vi "main.vi"() -> ()   [LabVIEW 2017]
uses:
  <vilib>/Instr/_visa.llb/VISA Set IO Buffer Mask.ctl
  <vilib>/Instr/_visa.llb/VISA Configure Serial Port (Instr).vi
  <vilib>/Analysis/NI_AALBase.lvlib
panel:
  in  "保存按钮":bool
  out "standard deviation":dbl caption="标准差" format="%#_2f"
  out "mean":dbl caption="均值" format="%#_7f"
  out "波形图表":dbl(graph)
  in  "配置Pcap":bool
  out "发送字符数":dbl
  in  "清空按钮":bool
  in  "timeout (10sec)":u32=100 caption="读取超时"
  in  "baud rate (9600)":u32=115200 caption="波特率"
  in  "VISA resource name":refnum<visa-resource-name> caption="串口号"
  in  "读取字节数":u32=1000
  out "未知的参数":string
  in  "参数数组":string[][](array[string])=[[""]]
  in  "发送自定义参数按钮":bool
  in  "自定义参数":string
  out "远程消息":string
  out "长度":i32=440
  out "连接状态":bool
  in  "查询次数":dbl
  in  "采集开关":bool
  in  "待处理数据":string
  # "最近10个数据统计值"
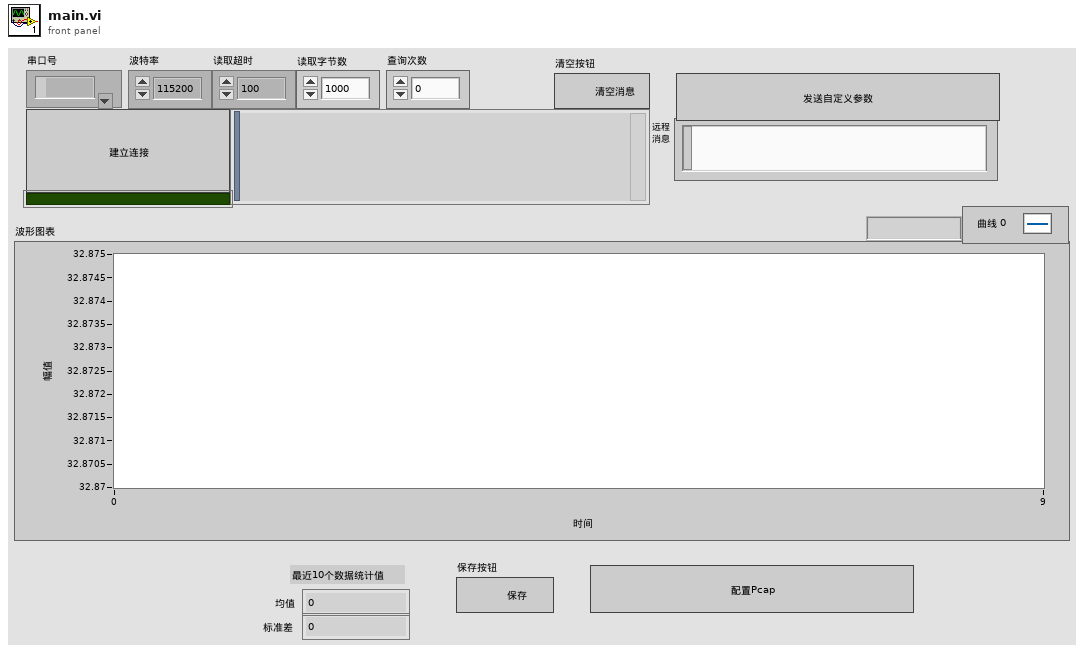
[diagram p1: front panel]
types:
  T1 = typedef "VISA Set IO Buffer Mask.ctl" = u16
  T2 = enum16{"big-endian, network order", "native, host order", "little-endian"}
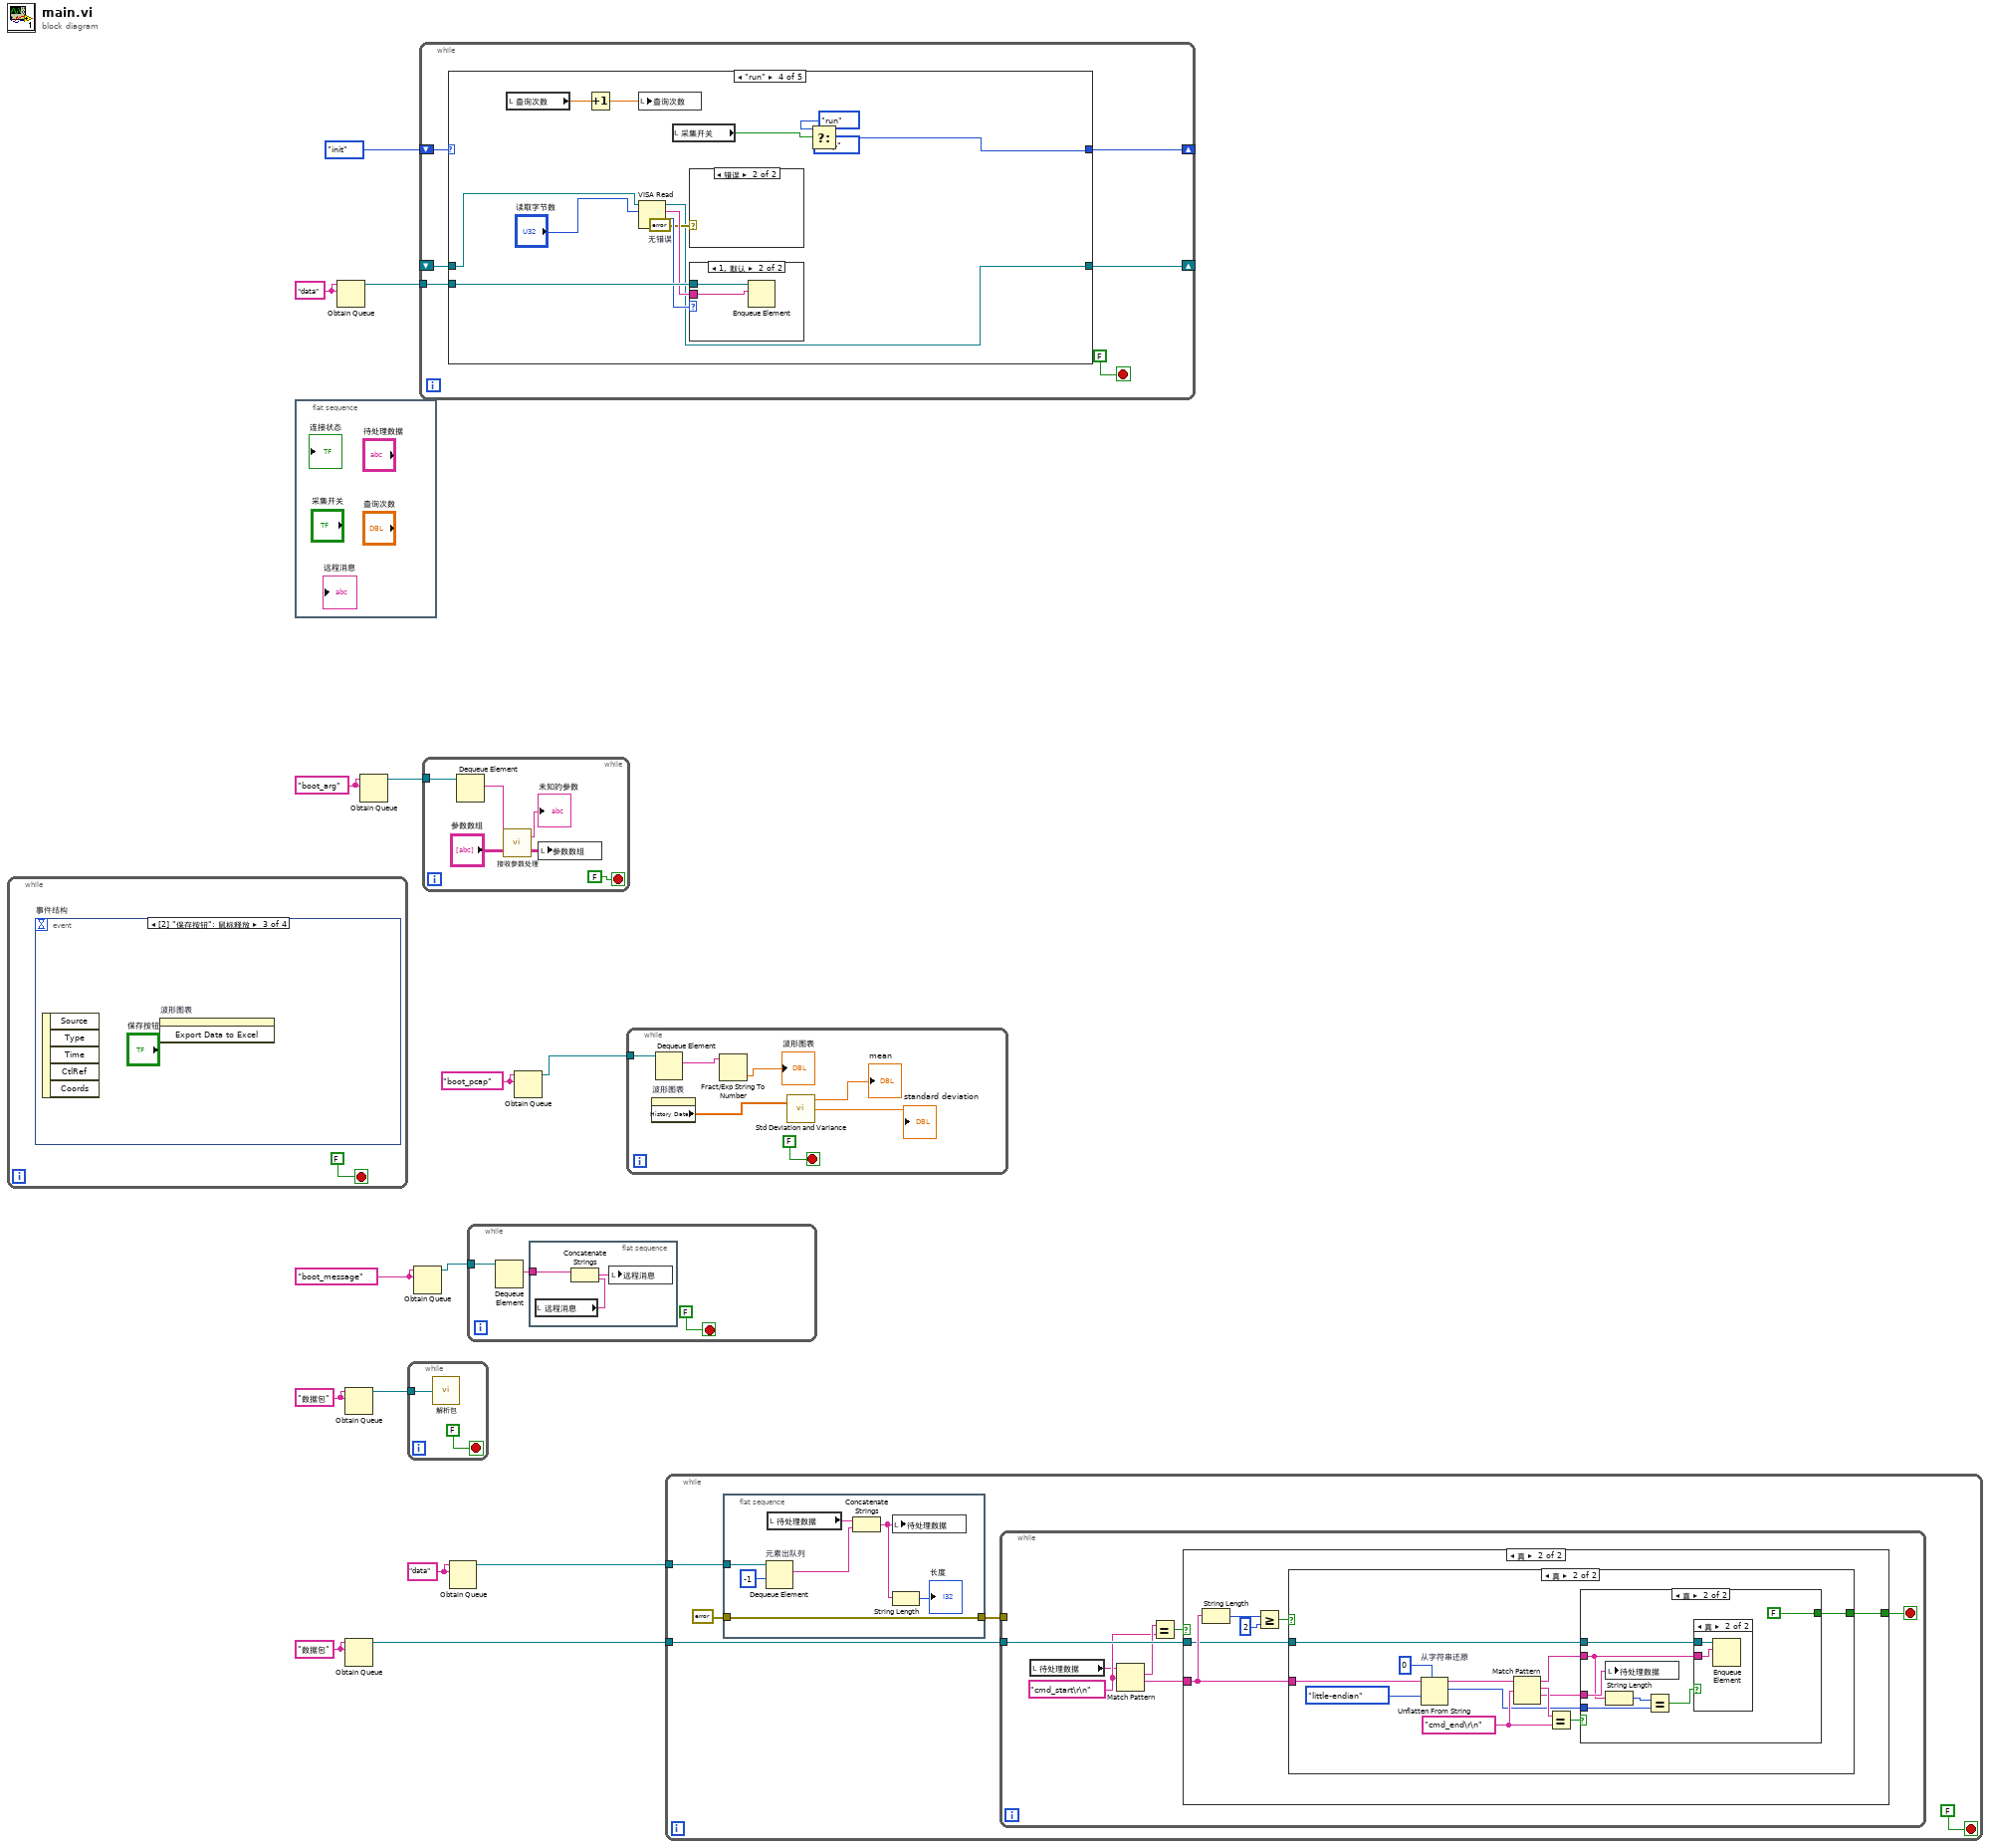
[diagram p0: block diagram]
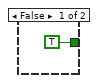
[diagram p2: hidden frame]
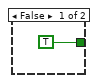
[diagram p3: hidden frame]
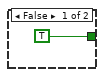
[diagram p4: hidden frame]
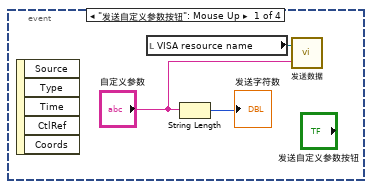
[diagram p6: hidden frame]
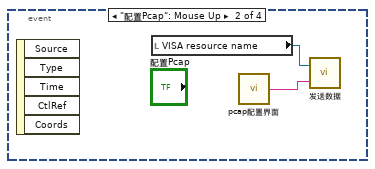
[diagram p7: hidden frame]
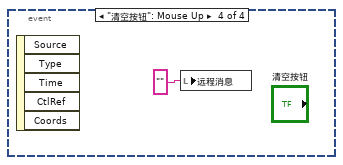
[diagram p8: hidden frame]
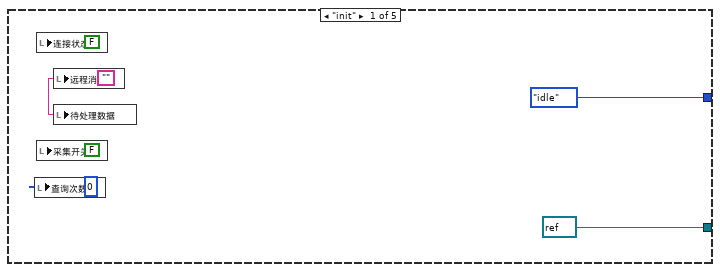
[diagram p9: hidden frame]
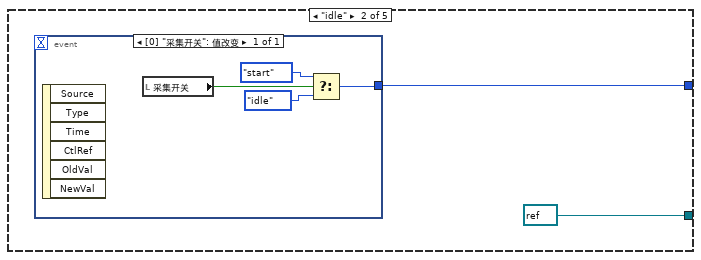
[diagram p10: hidden frame]
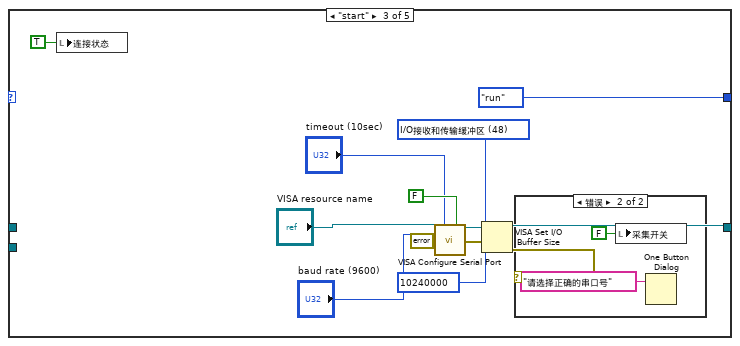
[diagram p11: hidden frame]
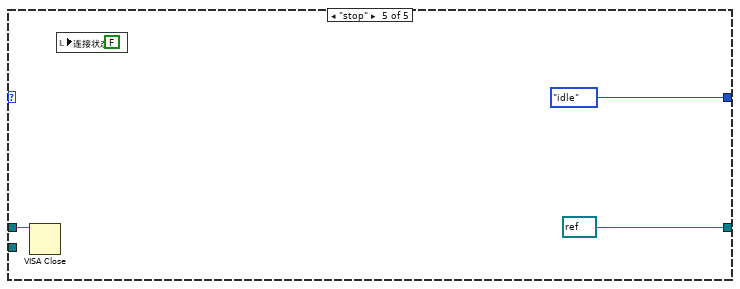
[diagram p15: hidden frame]
diagram:
  w2 = "boot_pcap" ("名称（未命名）")
  w4 = "boot_arg" ("名称（未命名）")
  w5 = "数据包" ("名称（未命名）")
  w8 = "boot_message" ("名称（未命名）")
  w11 = "数据包" ("名称（未命名）")
  w13 = "data" ("名称（未命名）")
  w15 = "data" ("名称（未命名）")
  n1 = while {
    stop <- FALSE stop-if-true
    n2 = event "事件结构" shown="[2] \"保存按钮\": 鼠标释放" {
      selector: _ -> [_ _ _ _]
      dyn-events: _ -> [_ _ _ _]
      timeout: _ -> [_ _ _ _]
      event "发送自定义参数按钮": Mouse Up {
        n3 = event-data() -> ()  [unwired: 1 in, 5 out]
        n4 = local read "VISA resource name"() -> (w19:refnum<visa-resource-name>)
        n5 = String Length(string="自定义参数") -> (length=→"发送字符数":i32)
        n6 = call "发送数据.vi"("发送数据"="自定义参数", "VISA资源名称"=w19) -> ()  [unwired: 1 in]
      }
      event "配置Pcap": Mouse Up {
        n7 = event-data() -> ()  [unwired: 1 in, 5 out]
        n8 = local read "VISA resource name"() -> (w20:refnum<visa-resource-name>)
        n9 = call "pcap配置界面.vi"() -> ("电子表格字符串"=w21:string)
        n10 = call "发送数据.vi"("发送数据"=w21, "VISA资源名称"=w20) -> ()  [unwired: 1 in]
      }
      event "保存按钮": Mouse Up {
        n11 = event-data() -> ()  [unwired: 1 in, 5 out]
        n12 = invoke on="波形图表" class="WFChart (严格)" method="Export Data to Excel"() -> ()  [unwired: 3 in, 3 out]
      }
      event "清空按钮": Mouse Up {
        n13 = event-data() -> ()  [unwired: 1 in, 5 out]
        n14 = local write "远程消息"("" ("远程消息")) -> ()
      }
    }
  }
  n15 = flat-sequence {
    frame #0 {
    }
  }
  n16 = Obtain Queue(name (unnamed)=w13, element data type=w13) -> (queue out=w12:refnum<queue>)  [unwired: 3 in, 2 out]
  n17 = Obtain Queue(name (unnamed)=w5, element data type=w5) -> (queue out=w6:refnum<queue>)  [unwired: 3 in, 2 out]
  n18 = Obtain Queue(name (unnamed)=w11, element data type=w11) -> (queue out=w10:refnum<queue>)  [unwired: 3 in, 2 out]
  n19 = Obtain Queue(name (unnamed)=w4, element data type=w4) -> (queue out=w3:refnum<queue>)  [unwired: 3 in, 2 out]
  n20 = while {
    tunnel: w6 -> [w23]
    stop <- FALSE stop-if-true
    n21 = call "解析包.vi"("数据包队列名称"=w23) -> ()  [unwired: 1 out]
  }
  n22 = Obtain Queue(name (unnamed)=w8, element data type=w8) -> (queue out=w7:refnum<queue>)  [unwired: 3 in, 2 out]
  n23 = while {
    shift-right: [w29] -> _
    shift-left: enum16{"start", "run", "stop", "idle", "init"}."init" -> [w30]
    tunnel: w12 -> [w27]
    shift-right: [w25] -> _
    shift-left: _ -> [w26]
    stop <- FALSE stop-if-true
    n24 = case shown="\"run\"" w30 {
      tunnel: [enum16{"start", "run", "stop", "idle", "init"}."idle" w38 enum16{"start", "run", "stop", "idle"}."run" w68 enum16{"start", "run", "stop", "idle"}."idle"] -> w29
      tunnel: w27 -> [_ _ _ w62 _]
      tunnel: [refnum<visa-resource-name> refnum ("VISA resource name out") refnum<visa-resource-name> refnum ("VISA resource name out") w47 w57 refnum<visa-resource-name> refnum ("VISA resource name out")] -> w25
      tunnel: w26 -> [_ _ _ w58 w74]
      frame "init" {
        w34 = ""
        n25 = local write "查询次数"(u16 0 ("宽")) -> ()
        n26 = local write "连接状态"(FALSE) -> ()
        n27 = local write "采集开关"(FALSE ("采样开关")) -> ()
        n28 = local write "远程消息"(w34) -> ()
        n29 = local write "待处理数据"(w34) -> ()
      }
      frame "idle" {
        n30 = event shown="[0] \"采集开关\": 值改变" {
          selector: _ -> [_]
          dyn-events: _ -> [_]
          timeout: _ -> [_]
          tunnel: [w39] -> w38
          event "采集开关": Value Change {
            n31 = event-data() -> ()  [unwired: 1 in, 6 out]
            n32 = local read "采集开关"() -> (w42:bool)
            n33 = Select(t=enum16{"start", "run", "stop", "idle"}."start", s=w42, f=enum16{"start", "run", "stop", "idle"}."idle") -> (s? t:f=w39:enum16{"start", "run", "stop", "idle"})
          }
        }
      }
      frame "start" {
        w46 = T1 48 items=["I/O接收缓冲区"=16, "I/O传输缓冲区"=32, "I/O接收和传输缓冲区"=48] ("Mask")
        n34 = local write "连接状态"(TRUE ("连接状态")) -> ()
        n35 = call-poly "VISA Configure Serial Port"("VISA resource name"="VISA resource name", "timeout (10sec)"="timeout (10sec)", "Enable Termination\nChar (T)"=FALSE ("Enable Termination\nChar (T)"), "baud rate (9600)"="baud rate (9600)") -> ("VISA resource name out"=w48:refnum<visa-resource-name>)  [unwired: 10 in, 1 out]
        n36 = VISA Set I/O Buffer Size(VISA resource name=w48, mask (16)=w46, size (4096)=u32 10240000 ("大小(4096)"), error in (no error)=errorcluster {"status"=FALSE, "code"=0, "source"=""} ("错误输入（无错误）")) -> (VISA resource name out=w47:refnum<visa-resource-name>, error out=w43:errorcluster)
        n37 = case shown="错误" w43 {
          frame No Error {
          }
          frame Error {
            n38 = local write "采集开关"(FALSE ("采集开关")) -> ()
            n39 = One Button Dialog(message="请选择正确的串口号" ("消息")) -> ()  [unwired: 1 in, 1 out]
          }
        }
      }
      frame "run" {
        w63 = errorcluster {"status"=FALSE, "code"=0, "source"=""}  # 无错误
        n40 = local read "查询次数"() -> (w66:dbl)
        n41 = Increment(x=w66) -> (x+1=w65:dbl)
        n42 = local write "查询次数"(w65) -> ()
        n43 = VISA Read(VISA resource name=w58, byte count="读取字节数", error in (no error)=w63) -> (VISA resource name out=w57:refnum<visa-resource-name>, read buffer=w61:string, return count=w60:u32, error out=w59:errorcluster)
        n44 = local read "采集开关"() -> (w70:bool)
        n45 = case shown="错误" w59 {
          frame No Error {
          }
          frame Error {
          }
        }
        n46 = case shown="1, 默认" w60 {
          tunnel: w62 -> [_ w71]
          tunnel: w61 -> [_ w72]
          frame 0 {
          }
          frame 1, Default {
            n47 = Enqueue Element(queue=w71, element=w72) -> ()  [unwired: 2 in, 3 out]
          }
        }
        n48 = Select(t=enum16{"start", "run", "stop", "idle"}."run", s=w70, f=enum16{"start", "run", "stop", "idle"}."stop") -> (s? t:f=w68:enum16{"start", "run", "stop", "idle"})
      }
      frame "stop" {
        n49 = VISA Close(VISA resource name=w74) -> ()  [unwired: 1 in, 1 out]
        n50 = local write "连接状态"(FALSE ("连接状态")) -> ()
      }
    }
  }
  n51 = while {
    tunnel: w3 -> [w82]
    stop <- FALSE stop-if-true
    n52 = Dequeue Element(queue=w82) -> (element=w77:string)  [unwired: 2 in, 3 out]
    n53 = call "接收参数处理.vi"("输入参数数组"="参数数组", "参数字符串"=w77) -> ("输出参数数组"=w80:string[][], "未知的参数"=→"未知的参数":string)
    n54 = local write "参数数组"(w80) -> ()
  }
  n55 = Obtain Queue(name (unnamed)=w15, element data type=w15) -> (queue out=w9:refnum<queue>)  [unwired: 3 in, 2 out]
  n56 = while {
    tunnel: w7 -> [w85]
    stop <- FALSE stop-if-true
    n57 = Dequeue Element(queue=w85) -> (element=w83:string)  [unwired: 2 in, 3 out]
    n58 = flat-sequence {
      tunnel: w83 -> [w86]
      frame #0 {
        n59 = local read "远程消息"() -> (w88:string)
        n60 = Concatenate Strings(w86, w88) -> (w87:string)
        n61 = local write "远程消息"(w87) -> ()
      }
    }
  }
  n62 = Obtain Queue(name (unnamed)=w2, element data type=w2) -> (queue out=w1:refnum<queue>)  [unwired: 3 in, 2 out]
  n63 = while {
    tunnel: w1 -> [w95]
    stop <- FALSE stop-if-true
    n64 = property on="波形图表" class="WFChart (严格)"() -> ("History Data"=w89:dbl[])  [unwired: 2 in, 2 out]
    n65 = Dequeue Element(queue=w95) -> (element=w93:string)  [unwired: 2 in, 3 out]
    n66 = Fract/Exp String To Number(string=w93) -> (number=→"波形图表":dbl)  [unwired: 3 in, 1 out]
    n67 = call <vilib>:"Std Deviation and Variance.vi"("X"=w89) -> ("mean"=→"mean":dbl, "standard deviation"=→"standard deviation":dbl)  [unwired: 1 in, 1 out]
  }
  n68 = while {
    tunnel: w10 -> [w99]
    tunnel: w9 -> [w98]
    stop <- FALSE stop-if-true
    n69 = flat-sequence {
      tunnel: w98 -> [w107]
      tunnel: errorcluster {"status"=FALSE, "code"=0, "source"=""} ("错误常量") -> [w101]
      tunnel: [w101] -> w96
      frame #0 {
        n70 = Dequeue Element "元素出队列"(queue=w107, timeout in ms (-1)=-1 ("超时毫秒(-1)")) -> (element=w105:string)  [unwired: 1 in, 3 out]
        n71 = local read "待处理数据"() -> (w104:string)
        n72 = Concatenate Strings(w104, w105) -> (w106:string)
        n73 = local write "待处理数据"(w106) -> ()
        n74 = String Length(string=w106) -> (length=→"长度":i32)
      }
    }
    n75 = while {
      tunnel: w99 -> [w112]
      tunnel: w96 -> [_]
      stop <- w108 stop-if-true
      w110 = "cmd_start\r\n" ("正则表达式")
      n76 = local read "待处理数据"() -> (w109:string)
      n77 = Match Pattern(string=w109, regular expression=w110) -> (match substring=w111:string, after substring=w113:string)  [unwired: 1 in, 2 out]
      n78 = Equal?(x=w111, y=w110) -> (x = y?=w114:bool)
      n79 = case shown="真" w114 {
        tunnel: w113 -> [_ w118]
        tunnel: w112 -> [_ w117]
        tunnel: [TRUE w116] -> w108
        frame False {
        }
        frame True {
          n80 = String Length(string=w118) -> (length=w121:i32)
          n81 = Greater Or Equal?(x=w121, y=2) -> (x >= y?=w119:bool)
          n82 = case shown="真" w119 {
            tunnel: w118 -> [_ w132]
            tunnel: w117 -> [_ w126]
            tunnel: [TRUE w124] -> w116
            frame False {
            }
            frame True {
              w129 = "cmd_end\r\n" ("结束码")
              n83 = Unflatten From String "从字符串还原"(type=u16 0, binary string=w132, byte order (0:big-endian, network order)=T2."little-endian" ("字节顺序(0:big-endian, network order)")) -> (rest of the binary string=w131:string, value=w123:u16)  [unwired: 2 in, 1 out]
              n84 = Match Pattern(string=w131, regular expression=w129) -> (before substring=w125:string, match substring=w130:string, after substring=w127:string)  [unwired: 1 in, 1 out]
              n85 = Equal?(x=w130, y=w129) -> (x = y?=w128:bool)
              n86 = case shown="真" w128 {
                tunnel: w127 -> [_ w142]
                tunnel: w126 -> [_ w140]
                tunnel: w125 -> [_ w137]
                tunnel: [TRUE FALSE] -> w124
                tunnel: w123 -> [_ w136]
                frame False {
                }
                frame True {
                  n87 = local write "待处理数据"(w142) -> ()
                  n88 = String Length(string=w137) -> (length=w138:i32)
                  n89 = Equal?(x=w138, y=w136) -> (x = y?=w141:bool)
                  n90 = case shown="真" w141 {
                    tunnel: w140 -> [_ w144]
                    tunnel: w137 -> [_ w143]
                    frame False {
                    }
                    frame True {
                      n91 = Enqueue Element(queue=w144, element=w143) -> ()  [unwired: 2 in, 3 out]
                    }
                  }
                }
              }
            }
          }
        }
      }
    }
  }
